vi "ResonanceAnalyzerJ&J.vi"() -> ()   [LabVIEW 2015]
panel:
  in  "stop":bool
  out "Resonance Curve":cluster{"all rows":dbl[], "Array":dbl[]}[](graph)
  in  "Tab Control":enum32{"Simulation", "Experiment"}(tab)
  in  "Input Parameter":T1
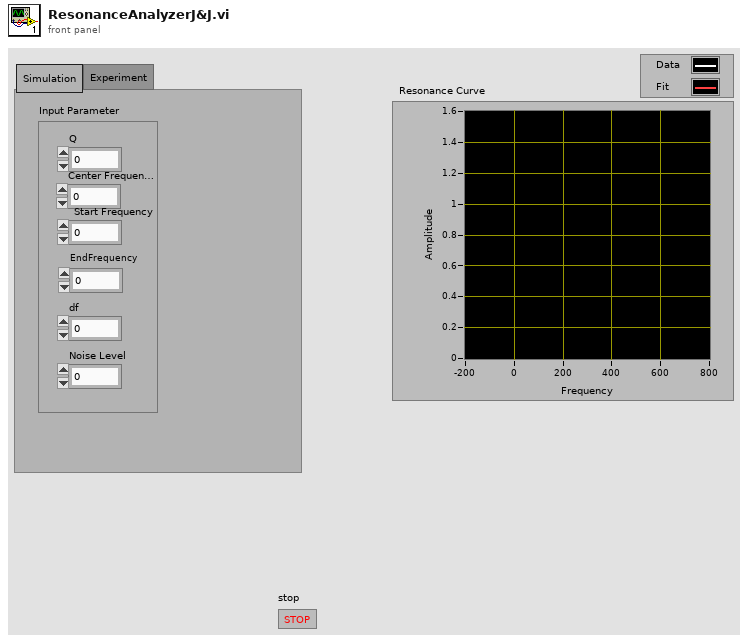
[diagram p1: front panel]
types:
  T1 = cluster{"Q":dbl, "Center Frequency":dbl, "Start Frequency":dbl, "EndFrequency":dbl, "df":dbl, "Noise Level":dbl}
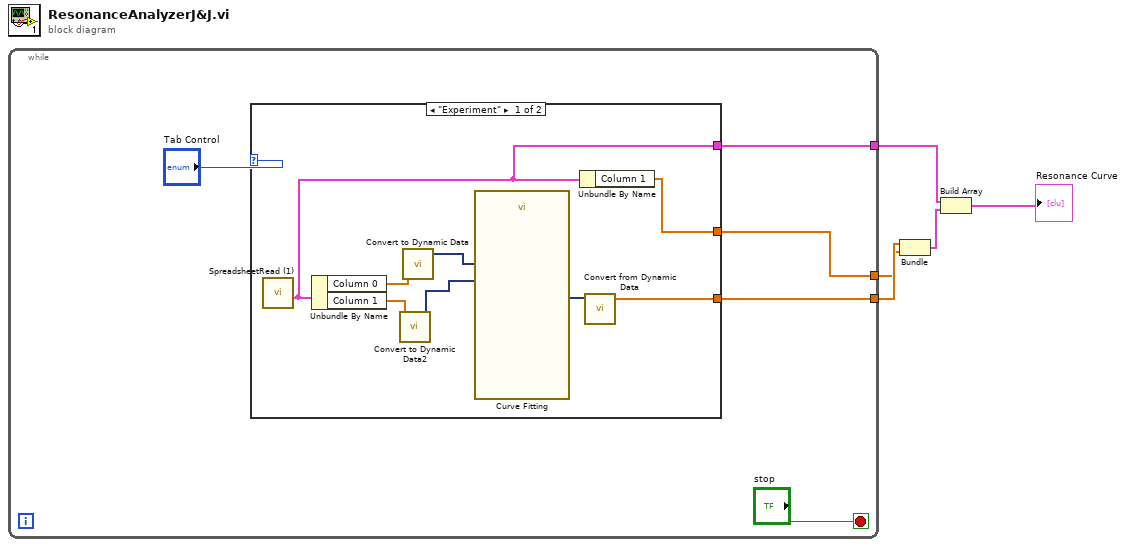
[diagram p0: block diagram]
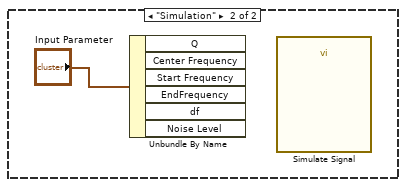
[diagram p2: hidden frame]
diagram:
  n1 = while {
    tunnel: [w8] -> w5
    tunnel: [w7] -> w1
    tunnel: [w6] -> w2
    stop <- "stop" stop-if-true
    n2 = case shown="\"Experiment\"" "Tab Control" {
      tunnel: [w14 _] -> w6
      tunnel: [w13 _] -> w7
      tunnel: [w12 _] -> w8
      frame "Experiment" {
        n3 = call "SpreadsheetRead (1).vi"() -> ("Output Cluster"=w12:cluster{"Column 0":dbl[], "Column 1":dbl[]})  [unwired: 10 in, 1 out]
        n4 = Unbundle By Name(w12) -> ("Column 0"=w16:dbl[], "Column 1"=w15:dbl[])
        n5 = call "Convert to Dynamic Data2"("Array"=w15) -> ("Dynamic Data Type"=w17:dynamicdata)  [unwired: 3 in]
        n6 = call "Convert to Dynamic Data"("Array"=w16) -> ("Dynamic Data Type"=w18:dynamicdata)  [unwired: 3 in]
        n7 = call "Curve Fitting"("Locations"=w18, "Signals"=w17) -> ("best fit"=w11:dynamicdata)  [unwired: 5 in, 4 out]
        n8 = Unbundle By Name(w12) -> ("Column 1"=w13:dbl[])
        n9 = call "Convert from Dynamic Data"("Dynamic Data Type"=w11) -> ("Array"=w14:dbl[])  [unwired: 3 in]
      }
      frame "Simulation" {
        n10 = Unbundle By Name("Input Parameter") -> ()  [unwired: 6 out]
        n11 = call "Simulate Signal"() -> ()  [unwired: 14 in, 2 out]
      }
    }
  }
  n12 = Bundle("Array"=w2, "Column 1"=w1) -> (w4:cluster{"Array":dbl[], "Column 1":dbl[]})  [unwired: 1 in]
  n13 = Build Array(w5, w4) -> (→"Resonance Curve":cluster{"Array":dbl[], "Column 1":dbl[]}[])
